vi "Tester.vi"() -> ()   [LabVIEW 2020, in "LoggerAPI.lvclass"]
uses:
  LoggerAPI.lvclass
  FileLogger/FileLogger.lvclass
  LogInfo/LogInfo.lvclass
  LogWarning/LogWarning.lvclass
  LogError/LogError.lvclass
  LogMessage/AbstractLogMessage.lvclass
  FileConfig/FileConfig.lvclass
  UILogger/UILogger.lvclass
  IResult/IResult.lvclass
  C:/Repo/LabVIEW-SOLID-Examples/Template-Logger/LogMessage/AbstractLogMessage.lvclass
  C:/Repo/LabVIEW-SOLID-Examples/Template-Logger/IAction/IAction.lvclass
  C:/Repo/LabVIEW-SOLID-Examples/Template-Logger/LogError/LogError.lvclass
  IConfig/IConfig.lvclass
  C:/Repo/LabVIEW-SOLID-Examples/Template-Logger/UILogger/UILogger.lvclass
  C:/Repo/LabVIEW-SOLID-Examples/Template-Logger/ILogger/ILogger.lvclass
panel:
  out "Timeout?":bool
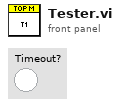
[diagram p1: front panel]
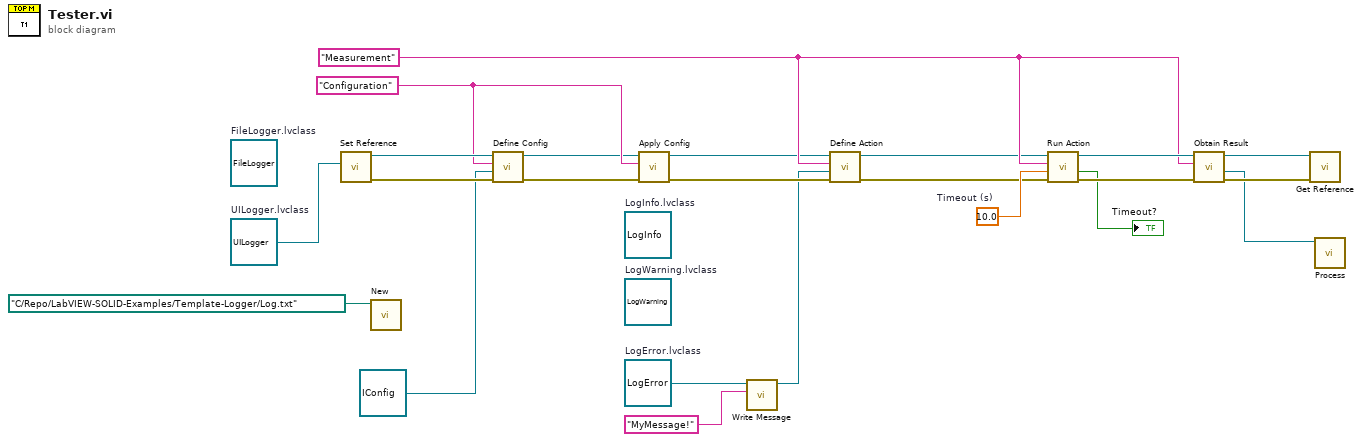
[diagram p0: block diagram]
diagram:
  w2 = refnum<class "UILogger.lvclass"> refnum  # UILogger.lvclass
  w7 = refnum<class "LogError.lvclass"> refnum  # LogError.lvclass
  (unwired) refnum<class "LogWarning.lvclass"> refnum  # LogWarning.lvclass
  (unwired) refnum<class "LogInfo.lvclass"> refnum  # LogInfo.lvclass
  (unwired) refnum<class "FileLogger.lvclass"> refnum  # FileLogger.lvclass
  w18 = 10.0  # Timeout (s)
  w17 = "Measurement" ("Name")
  w22 = "Configuration" ("Name")
  n1 = call "Set Reference.vi"("Reference"=w2) -> ("Error Out"=w21:errorcluster, "Logger Out"=w23:refnum<class "LoggerAPI.lvclass">)  [unwired: 9 in]
  n2 = call "New.vi"("File Path"=path "C:/Repo/LabVIEW-SOLID-Examples/Template-Logger/Log.txt") -> ()  [unwired: 10 in, 1 out]
  n3 = call "Define Config.vi"("Error In"=w21, "Config"=refnum<class "IConfig.lvclass"> refnum ("IConfig.lvclass"), "Name"=w22, "Logger In"=w23) -> ("Error Out"=w15:errorcluster, "Logger Out"=w16:refnum<class "LoggerAPI.lvclass">)  [unwired: 6 in]
  n4 = call "Apply Config.vi"("ErrorIn"=w15, "Name"=w22, "TopModuleIn"=w16) -> ("ErrorOut"=w13:errorcluster, "TopModuleOut"=w14:refnum<class "LoggerAPI.lvclass">)  [unwired: 7 in]
  n5 = call "Write Message.vi"("Message"="MyMessage!", "LogMessage In"=w7) -> ("LogMessage Out"=w6:refnum<class "LogError.lvclass">)  [unwired: 9 in]
  n6 = call "Define Action.vi"("Error In"=w13, "Measurement"=w6, "Name"=w17, "Logger In"=w14) -> ("Error Out"=w11:errorcluster, "Logger Out"=w12:refnum<class "LoggerAPI.lvclass">)  [unwired: 6 in]
  n7 = call "Run Action.vi"("Error In"=w11, "Timeout (s)"=w18, "Action"=w17, "Logger In"=w12) -> ("Error Out"=w19:errorcluster, "Timeout?"=→"Timeout?":bool, "Logger Out"=w20:refnum<class "LoggerAPI.lvclass">)  [unwired: 5 in]
  n8 = call "Obtain Result.vi"("Error In"=w19, "Name"=w17, "Logger In"=w20) -> ("Error Out"=w4:errorcluster, "Result Out"=w3:refnum<class "IResult.lvclass">, "Logger Out"=w5:refnum<class "LoggerAPI.lvclass">)  [unwired: 5 in, 1 out]
  n9 = call "Get Reference.vi"("Error In"=w4, "Logger In"=w5) -> ()  [unwired: 7 in, 3 out]
  n10 = call-dynamic "Process.vi"("IResult In"=w3) -> ()  [unwired: 9 in, 2 out]
